vi "Depth Parameters to Array.vi"(11 "Roughness Parameters in":T1) -> (3 "Array":dbl[](array[numeric]))   [LabVIEW 2018]
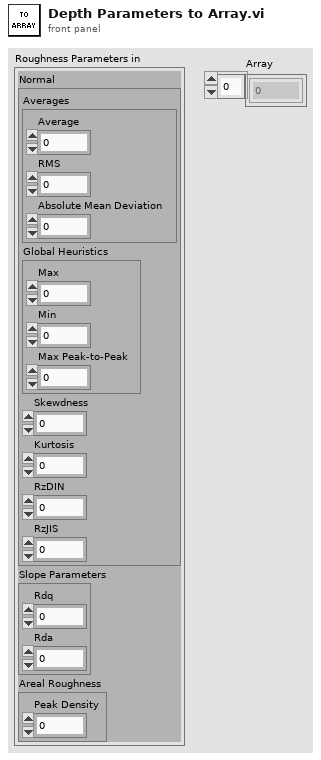
[diagram p1: front panel]
types:
  T1 = cluster{"Normal":cluster{"Averages":cluster{"Average":dbl, "RMS":dbl, "Absolute Mean Deviation":dbl}, "Global Heuristics":cluster{"Max":dbl, "Min":dbl, "Max Peak-to-Peak":dbl}, "Skewdness":dbl, "Kurtosis":dbl, "RzDIN":dbl, "RzJIS":dbl}, "Slope Parameters":cluster{"Rdq":dbl, "Rda":dbl}, "Areal Roughness":cluster{"Peak Density":dbl}}
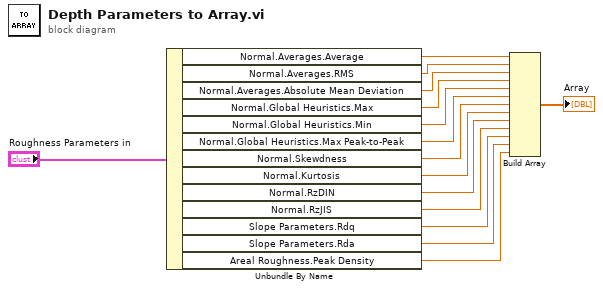
[diagram p0: block diagram]
diagram:
  n1 = Unbundle By Name("Roughness Parameters in") -> ("Normal.Averages.Average"=w3:dbl, "Normal.Averages.RMS"=w4:dbl, "Normal.Averages.Absolute Mean Deviation"=w5:dbl, "Normal.Global Heuristics.Max"=w6:dbl, "Normal.Global Heuristics.Min"=w7:dbl, "Normal.Global Heuristics.Max Peak-to-Peak"=w8:dbl, "Normal.Skewdness"=w9:dbl, "Normal.Kurtosis"=w10:dbl, "Normal.RzDIN"=w11:dbl, "Normal.RzJIS"=w12:dbl, "Slope Parameters.Rdq"=w13:dbl, "Slope Parameters.Rda"=w14:dbl, "Areal Roughness.Peak Density"=w15:dbl)
  n2 = Build Array(w3, w4, w5, w6, w7, w8, w9, w10, w11, w12, w13, w14, w15) -> (→"Array":dbl[])
